vi "GET Slope.vi"() -> (0 "Slope":dbl)   [LabVIEW 2013]
doc: "Get the current slope value. Slope units are nm/V."
uses:
  Action.ctl
  Calibration Output FGV Selector.ctl
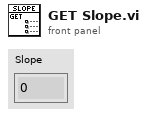
[diagram p1: front panel]
types:
  T1 = typedef "Calibration Output FGV Selector.ctl" = enum16{"X Constant", "Y Constant", "Z Constant", "Power Peak", "Slope", "Spring Constant"}
  T2 = typedef "Action.ctl" = enum16{"GET", "PUT", "DELETE"}
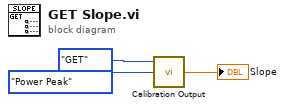
[diagram p0: block diagram]
diagram:
  n1 = call "Calibration Output.vi"("Calibration Output FGV Selector"=Calibration_Output_FGV_Selector."Power Peak", "Action"=Action."GET") -> ("Output"=→"Slope":dbl)  [unwired: 1 in]
